vi "SwerveChooseBestAngle.vi"(5 "Goal Override":bool, 7 "Goal Override Angle (deg) [-180,+180]":dbl format="%#_13g", 8 "Hysteresis (deg)":dbl=10.0 format="%#_13g", 10 "Goal Angle (deg) [-180,+180]":dbl format="%#_13g", 11 "Current Angle (deg) [-180,+180]":dbl format="%#_13g") -> (0 "Invert Speed  Motor (?)":bool, 2 "Angular Distance (deg)":dbl format="%_4g")   [LabVIEW 2019]
doc: "Based on the Current Angle and the Goal Angle, this VI calulates the signed angular distance. Taking into account the option to invert the direction of the swerve drive motor and always picking the shortest travel distance. The hysteresis prevents undesirable vacillation between angle choices."
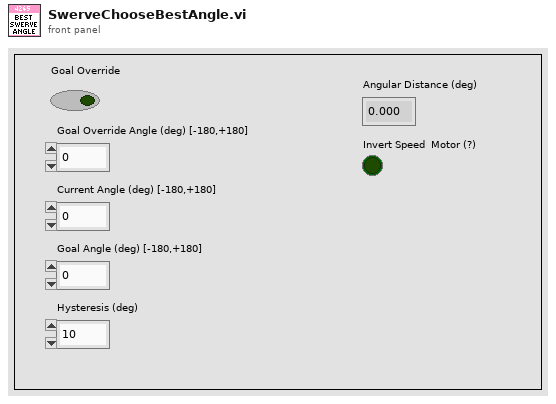
[diagram p1: front panel]
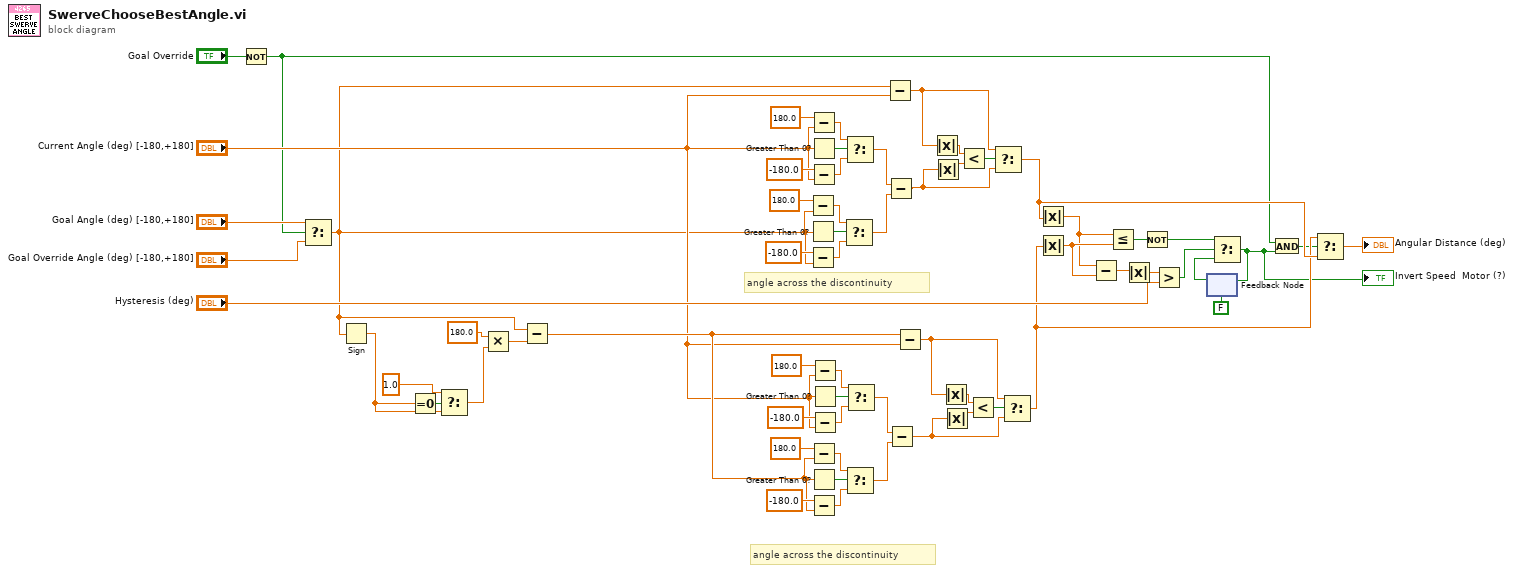
[diagram p0: block diagram]
diagram:
  # "angle across the discontinuity"
  # "angle across the discontinuity"
  n1 = Not(x="Goal Override") -> (.not. x?=w2:bool)
  n2 = Select(t="Goal Angle (deg) [-180,+180]", s=w2, f="Goal Override Angle (deg) [-180,+180]") -> (s? t:f=w4:dbl)
  n3 = Sign(1:w4) -> (0:w13:dbl)
  n4 = Equal To 0?(x=w13) -> (x = 0?=w14:bool)
  n5 = Select(t=1.0, s=w14, f=w13) -> (s? t:f=w10:dbl)
  n6 = Multiply(x=180.0 ("y"), y=w10) -> (x*y=w62:dbl)
  n7 = Subtract(x=w4, y=w62) -> (x-y=w35:dbl)
  n8 = Subtract(x=180.0, y=w4) -> (x-y=w23:dbl)
  n9 = Greater Than 0?(x=w4) -> (x > 0?=w25:bool)
  n10 = Subtract(x=-180.0, y=w4) -> (x-y=w21:dbl)
  n11 = Subtract(x=180.0, y="Current Angle (deg) [-180,+180]") -> (x-y=w28:dbl)
  n12 = Greater Than 0?(x="Current Angle (deg) [-180,+180]") -> (x > 0?=w30:bool)
  n13 = Subtract(x=-180.0, y="Current Angle (deg) [-180,+180]") -> (x-y=w26:dbl)
  n14 = Subtract(x=180.0, y=w35) -> (x-y=w44:dbl)
  n15 = Greater Than 0?(x=w35) -> (x > 0?=w46:bool)
  n16 = Subtract(x=-180.0, y=w35) -> (x-y=w42:dbl)
  n17 = Subtract(x=180.0, y="Current Angle (deg) [-180,+180]") -> (x-y=w50:dbl)
  n18 = Greater Than 0?(x="Current Angle (deg) [-180,+180]") -> (x > 0?=w52:bool)
  n19 = Subtract(x=-180.0, y="Current Angle (deg) [-180,+180]") -> (x-y=w48:dbl)
  n20 = Select(t=w23, s=w25, f=w21) -> (s? t:f=w19:dbl)
  n21 = Select(t=w28, s=w30, f=w26) -> (s? t:f=w20:dbl)
  n22 = Select(t=w44, s=w46, f=w42) -> (s? t:f=w40:dbl)
  n23 = Select(t=w50, s=w52, f=w48) -> (s? t:f=w41:dbl)
  n24 = Subtract(x=w4, y="Current Angle (deg) [-180,+180]") -> (x-y=w31:dbl)
  n25 = Subtract(x=w20, y=w19) -> (x-y=w17:dbl)
  n26 = Subtract(x=w41, y=w40) -> (x-y=w39:dbl)
  n27 = Subtract(x=w35, y="Current Angle (deg) [-180,+180]") -> (x-y=w36:dbl)
  n28 = Absolute Value(x=w31) -> (abs(x)=w32:dbl)
  n29 = Absolute Value(x=w17) -> (abs(x)=w33:dbl)
  n30 = Absolute Value(x=w36) -> (abs(x)=w37:dbl)
  n31 = Absolute Value(x=w39) -> (abs(x)=w38:dbl)
  n32 = Less?(x=w32, y=w33) -> (x < y?=w34:bool)
  n33 = Less?(x=w37, y=w38) -> (x < y?=w47:bool)
  n34 = Select(t=w31, s=w34, f=w17) -> (s? t:f=w9:dbl)
  n35 = Select(t=w36, s=w47, f=w39) -> (s? t:f=w8:dbl)
  n36 = Absolute Value(x=w9) -> (abs(x)=w53:dbl)
  n37 = Absolute Value(x=w8) -> (abs(x)=w54:dbl)
  n38 = Subtract(x=w53, y=w54) -> (x-y=w58:dbl)
  n39 = Less Or Equal?(x=w53, y=w54) -> (x <= y?=w16:bool)
  n40 = Absolute Value(x=w58) -> (abs(x)=w57:dbl)
  n41 = Not(x=w16) -> (.not. x?=w15:bool)
  n42 = Greater?(x=w57, y="Hysteresis (deg)") -> (0:w55:bool)
  n43 = feedback #1(FALSE) -> (w60:bool)
  n44 = Select(t=w15, s=w55, f=w60) -> (s? t:f=w6:bool)
  "Invert Speed  Motor (?)" <- w6
  n45 = feedback-in #1(w6) -> ()
  n46 = And(x=w2, y=w6) -> (x .and. y?=w7:bool)
  n47 = Select(t=w8, s=w7, f=w9) -> (s? t:f=→"Angular Distance (deg)":dbl)
